vi "Elevator Encoder Read.vi"(9 "Reset?":bool) -> (1 "Height":dbl)   [LabVIEW 2017]
uses:
  Common Code/Elevator Encoder Values.ctl
  Robot Global Data.vi
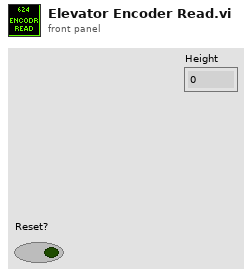
[diagram p1: front panel]
types:
  T1 = typedef "Elevator Encoder Values.ctl" = cluster{"Encoder Values":cluster{"Distance":dbl, "Speed":dbl, "Tick":dbl}}
  T2 = typedef "Dashboard Control Data.ctl" = cluster{"Drivetrain Settings Cluster":T3, "Intake Presets":T5, "Elevator Settings Cluster":T6, "Drivetrain Encoder Values":T8, "Auton Chooser":T9, "Auton Presets":cluster{"Start Position":dbl}, "Elevator Encoder Values":T1}
  T3 = typedef "Drivetrain Settings Cluster.ctl" = cluster{"Gyro Steer PID Gains":T4, "Distance Drive PID Gains":T4, "Drive Tolerance":dbl, "Gyro Tolerance":dbl, "Gyro Output":dbl, "Distance Output":dbl, "Y Power Multiplier":dbl, "Turn Power Multiplier":dbl, "Creep Rate":dbl, "Encoder Reset":bool, "DT Mode Modifier":enum16{"None, Default", "Cube", "Square"}, "Left Encoder Tick Constant":dbl, "Right Encoder Tick Constant":dbl, "Shift Speed":dbl, "Zero Gyro":bool}
  T4 = typedef "PID Gains Cluster.ctl" = cluster{"Integral Time":dbl, "Proportional Gain":dbl, "Derivative Time":dbl}
  T5 = typedef "Intake Presets.ctl" = cluster{"Idle Angle":dbl, "Mid Angle":dbl, "Low Angle":dbl, "Outtake Power":dbl, "Intake Power":dbl, "Unstuck":dbl, "Angle Tolerance":dbl, "Max Angle":dbl, "Max Current":dbl, "Current Trip Time":dbl, "Reset Encoder?":bool, "Encoder Scale":dbl, "PID gains":cluster{"proportional gain (Kc)":dbl, "integral time (Ti, min)":dbl, "derivative time (Td, min)":dbl}, "output range":cluster{"output high":dbl, "output low":dbl}, "IR Constant Pull Rate":dbl}
  T6 = typedef "Elevator Settings Cluster.ctl" = cluster{"Ground Height":dbl, "Switch Height":dbl, "Scale High Height ":dbl, "Scale Low Height":dbl, "Elevator PID Gains":T7, "Elevator Tolerance":dbl, "Reset Encoders":bool, "Encoder Scale":dbl, "Max Height":dbl, "Mid Height":dbl, "output range":cluster{"output high":dbl, "output low":dbl}, "Slow Down Tolerance":dbl, "Tick Constant":dbl, "Anti-tip Multiplier":dbl}
  T7 = typedef "PID Gains.ctl" = cluster{"proportional gain (Kc)":dbl, "integral time (Ti, min)":dbl, "derivative time (Td, min)":dbl}
  T8 = typedef "DT Encoder Values.ctl" = cluster{"Left Encoder":cluster{"Distance":dbl, "Speed":dbl, "Tick":dbl}, "Right Encoder":cluster{"Distance":dbl, "Speed":dbl, "Tick":dbl}}
  T9 = typedef "Auton Chooser.ctl" = cluster{"Left":bool, "Center":bool, "Right":bool, "Scale":bool, "Both":bool, "Switch":bool}
  T10 = typedef "WPI_EncoderDevRef.ctl" = cluster{"DevStatus":errorcluster, "EncoderIndex":T11, "CounterIndex":T12, "DistancePerCount":dbl, "Decoding Type":T13}
  T11 = typedef "FPGA_EncoderIdx.ctl" = enum8{"Enc 0", "Enc 1", "Enc 2", "Enc 3", "Enc 4", "Enc 5", "Enc 6", "Enc 7", "Invalid"}
  T12 = typedef "FPGA_CounterCtrSystemIndex.ctl" = enum8{"Ctr 0", "Ctr 1", "Ctr 2", "Ctr 3", "Ctr 4", "Ctr 5", "Ctr 6", "Ctr 7", "Invalid"}
  T13 = typedef "WPI_EncoderType.ctl" = enum16{"1x", "2x", "4x"}
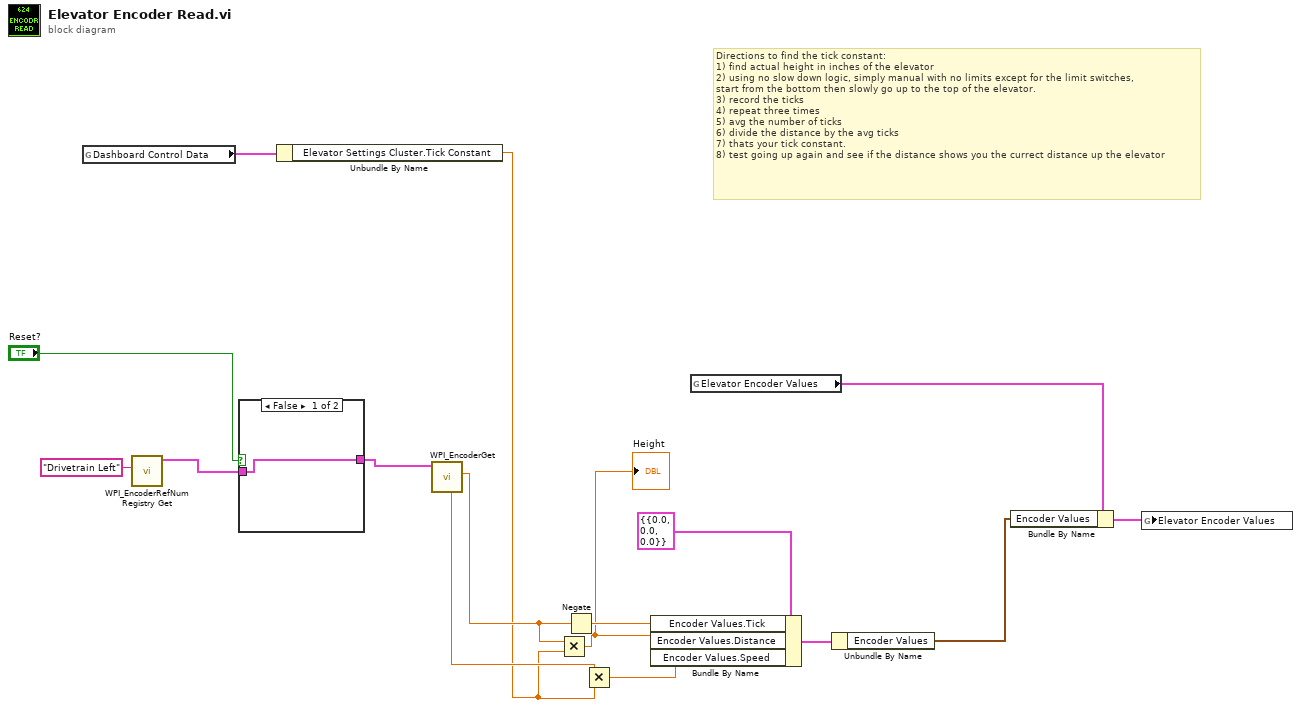
[diagram p0: block diagram]
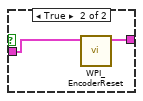
[diagram p2: hidden frame]
diagram:
  # "Directions to find the tick constant: \n1) find actual height in inches of the elevator\n2) using no slow down logic, simply manual with no limits except for the limit switches,\nstart from the bottom then slowly go up to the top of the elevator.\n3) record the ticks\n4) repeat three times\n5) avg the number of ticks\n6) divide the distance by the avg ticks\n7) thats your tick constant. \n8) test going up again and see if the distance shows you the currect distance up the elevator"
  n1 = global read "Robot Global Data.vi" "Dashboard Control Data"() -> (w12:T2)
  n2 = call <vilib>:"WPI_EncoderRefNum Registry Get.vi"("refnum name"="Drivetrain Left") -> ("EncoderDevRef"=w14:T10)  [unwired: 9 in, 1 out]
  n3 = case shown="False" "Reset?" {
    tunnel: w14 -> [w17 w19]
    tunnel: [w17 w18] -> w13
    frame False {
    }
    frame True {
      n4 = call <vilib>:"WPI_EncoderReset.vi"("EncoderDevRef"=w19) -> ("EncoderDevRef"=w18:T10)  [unwired: 9 in, 1 out]
    }
  }
  n5 = Unbundle By Name(w12) -> ("Elevator Settings Cluster.Tick Constant"=w4:dbl)
  n6 = call <vilib>:"WPI_EncoderGet.vi"("EncoderDevRef"=w13) -> ("Distance"=w6:dbl, "Rate"=w5:dbl)  [unwired: 5 in, 4 out]
  n7 = Multiply(x=w6, y=w4) -> (x*y=w1:dbl)
  "Height" <- w1
  n8 = Negate(x=w6) -> (-x=w9:dbl)
  n9 = Multiply(x=w5, y=w4) -> (x*y=w8:dbl)
  n10 = Bundle By Name(cluster=T1 {"Encoder Values"={"Distance"=0.0, "Speed"=0.0, "Tick"=0.0}} ("Elevator Encoder Values"), "Encoder Values.Tick"=w9, "Encoder Values.Distance"=w1, "Encoder Values.Speed"=w8) -> (w3:T1)
  n11 = global read "Robot Global Data.vi" "Elevator Encoder Values"() -> (w11:T1)
  n12 = Unbundle By Name(w3) -> ("Encoder Values"=w2:cluster{"Distance":dbl, "Speed":dbl, "Tick":dbl})
  n13 = Bundle By Name(cluster=w11, "Encoder Values"=w2) -> (w10:T1)
  n14 = global write "Robot Global Data.vi" "Elevator Encoder Values"(w10) -> ()
